vi "Page_Source_Settings_Validate_Top_Level_Inclusion.vi"(8 "error in (no error)":errorcluster, 9 "sourceInclusion in":T1=enum."Include", 10 "AB_Source in":refnum<class "AB_Source.lvclass">, 11 "AB_Build in":refnum<class "AB_Build.lvclass">) -> (0 "error out":errorcluster, 1 "sourceInclusion out":T1=enum."Include", 3 "AB_Build out":refnum<class "AB_Build.lvclass">)   [LabVIEW 2020, in "AB_Build.lvclass"]
uses:
  <vilib>/AppBuilder/AB_Classes/Build/AB_Build.lvclass
  <vilib>/AppBuilder/AB_Classes/Source/AB_Source.lvclass
  <vilib>/AppBuilder/AB_Source_Inclusion.ctl
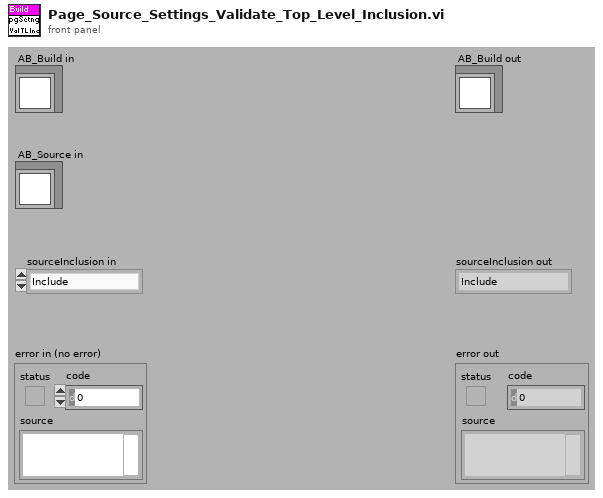
[diagram p1: front panel]
types:
  T1 = typedef "AB_Source_Inclusion.ctl" = enum16{"IncludeIfReferenced", "Include", "Exclude", "TopLevel"}
  T2 = typedef "AB_Build.ctl" = cluster{"buildSpecName":string, "buildSpecDescription":string, "destinations":refnum<class "AB_Destination.lvclass">[], "exclusionOption":T3, "defaultLanguage":string, "supportedLanguages":string[], "excludedDirectories":path[], "buildContext":refnum<vi>, "buildObject":T4, "preview":bool, "programatic":bool, "progressBarEvents":T5, "userLog_Path":path, "preActionID":string, "preAction_Path":path, "postActionID":string, "postAction_Path":path, "eng_checkForBrokenVIs?":bool, "eng_verboseLinkerErrors?":bool, "localDest_Path":path, "targetDest_Path":path, "removeVIObject":u16, "cache":refnum<class "PreviewCache.lvclass">, "use cache":bool, "previewCache_ID":string, "buildCache_ID":string, "eng_TempLocalDest_Path":path, "eng_collectDependencies?":bool, "versionInfo":cluster{"buildVersion":cluster{"major":u16, "minor":u16, "patch":u16, "build":u16}, "autoIncrement":bool}, "eng_enableVIChecksums":bool}
  T3 = typedef "AB_Exclusion_Option.ctl" = cluster{"typedefs":bool, "polymorphicVIs":bool, "unusedLibraryItems":bool, "modifyLibraryFile":bool, "edit-timeDependencies":bool, "inlineVIs":bool, "dependent PPLs":bool, "dependent DLLs":bool}
  T4 = typedef "ItemRef.ctl" = u64
  T5 = typedef "provcom_ProgressBar_Events.ctl" = cluster{"newJob":refnum<user-event>, "newItem":refnum<user-event>, "errorMsg":T6, "cancel":refnum<user-event>}
  T6 = typedef "mxLvBuildError.ctl" = refnum<user-event>
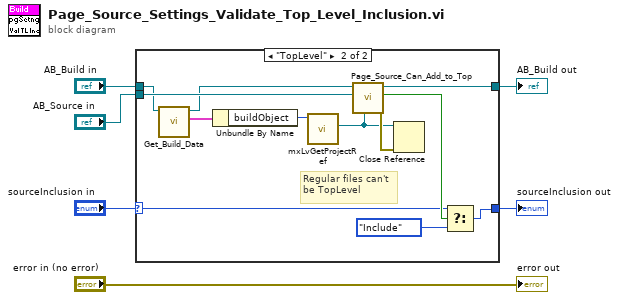
[diagram p0: block diagram]
diagram:
  n1 = case shown="\"TopLevel\"" "sourceInclusion in" {
    selector: "sourceInclusion in" -> [w7 w15]
    tunnel: "AB_Build in" -> [w8 w12]
    tunnel: [w8 w18] -> w4
    tunnel: "AB_Source in" -> [_ w17]
    tunnel: [w7 w16] -> w2
    frame Default {
    }
    frame "TopLevel" {
      # "Regular files can't be TopLevel"
      n2 = call <vilib>:"Get_Build_Data.vi"("Class in"=w12) -> ("data"=w13:T2, "Class out"=w11:refnum<class "AB_Build.lvclass">)  [unwired: 1 in, 8 out]
      n3 = Unbundle By Name(w13) -> ("buildObject"=w14:T4)
      n4 = call <resource>:"mxLvGetProjectRef.vi"("Item"=w14) -> ("Project Refnum"=w9:refnum<vi>)  [unwired: 1 in, 9 out]
      n5 = call-dynamic "Page_Source_Can_Add_to_Top.vi"("Project Refnum"=w9, "AB_Source in"=w17, "AB_Build in"=w11) -> ("error out"=w10:errorcluster, "canAddToTop"=w20:bool, "AB_Build out"=w18:refnum<class "AB_Build.lvclass">)  [unwired: 5 in, 1 out]
      n6 = Close Reference(reference=w9, error in (no error)=w10) -> ()  [unwired: 1 out]
      n7 = Select(t=w15, s=w20, f=AB_Source_Inclusion."Include" ("sourceInclusion")) -> (s? t:f=w16:T1)
    }
  }
  "AB_Build out" <- w4
  "sourceInclusion out" <- w2
  "error out" <- "error in (no error)"
